vi "Read Child Attributes Map.vi"(7 "Actor in":refnum<class "Actor.lvclass">) -> (2 "Child Attributes Map":T1)   [LabVIEW 2020, in "jettl.lvlib" / "Actor Specific.lvlib"]
uses:
  Actor Specific.lvlib
  Actor/Actor.lvclass
  Transport/Transport.lvclass
  Actor Attributes.ctl
  jettl.lvlib
  Child Actor Attributes Map.ctl
  Msg/Msg.lvclass
  Msgs.ctl
  Msg Names.ctl
  Unified Layer.ctl
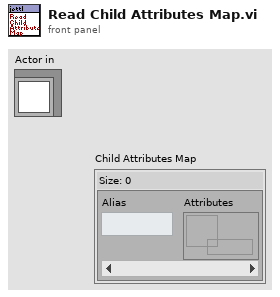
[diagram p1: front panel]
types:
  T1 = typedef "jettl.lvlib/Child Actor Attributes Map.ctl" = map{string, refnum<data-value>}
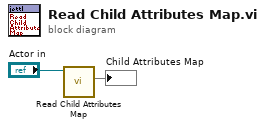
[diagram p0: block diagram]
diagram:
  n1 = call-dynamic "Read Child Attributes Map.vi"("Actor in"="Actor in") -> ("Child Attributes Map"=→"Child Attributes Map":T1)  [unwired: 10 in]
